vi "Convert Boolean to Floor.vi"(8 "error in (no error)":errorcluster, 11 "Boolean array":bool[](array[boolean])) -> (0 "error out":errorcluster, 1 "number":u32, 3 "Floor Number":i32)   [LabVIEW 2018]
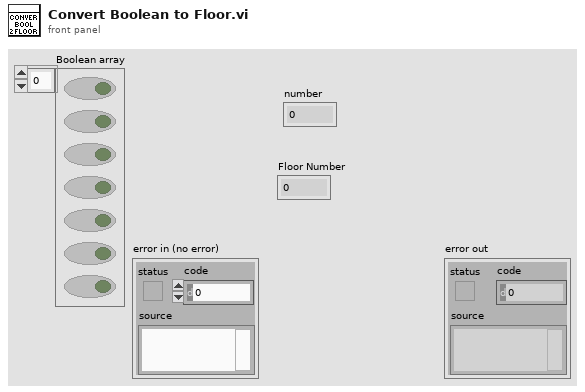
[diagram p1: front panel]
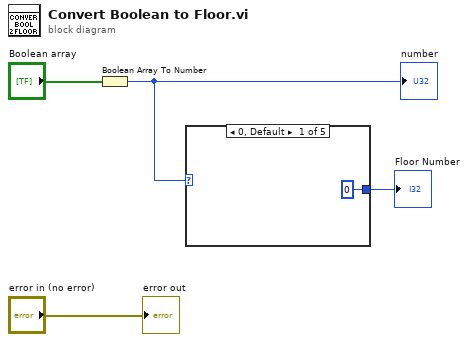
[diagram p0: block diagram]
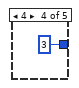
[diagram p4: hidden frame]
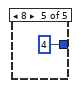
[diagram p5: hidden frame]
diagram:
  n1 = Boolean Array To Number(Boolean array="Boolean array") -> (number=w4:u32)
  "number" <- w4
  n2 = case shown="0, Default" w4 {
    selector: w4 -> [_ w6 w7 _ _]
    tunnel: [u32 0 w6 w7 u32 3 u32 4] -> w3
    frame 0, Default {
    }
    frame 1 {
    }
    frame 2 {
    }
    frame 4 {
    }
    frame 8 {
    }
  }
  "Floor Number" <- w3
  "error out" <- "error in (no error)"
